vi "DAQmxTaskInfo.vi"(0 "task in":refnum<k21>) -> (1 "ChanType":i32, 2 "Name":refnum<k21>)   [LabVIEW 2010]
uses:
  Program Files/National Instruments/LabVIEW 2010/resource/objmgr/daqmx.rc
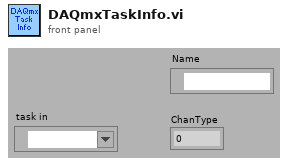
[diagram p1: front panel]
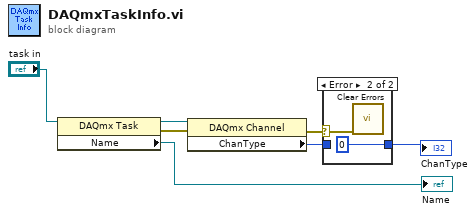
[diagram p0: block diagram]
diagram:
  n1 = property class="DAQmx Task"(reference="task in") -> (reference out=w3:refnum<k21>, error out=w1:errorcluster, "Name"=→"Name":refnum<k21>)  [unwired: 1 in]
  n2 = property class="DAQmx Channel"(reference=w3, error in=w1) -> (error out=w5:errorcluster, "ChanType"=w6:i32)  [unwired: 1 out]
  n3 = case shown="Error" w5 {
    selector: w5 -> [_ w10]
    tunnel: w6 -> [w8 _]
    tunnel: [w8 0 ("ChanType")] -> w7
    frame No Error {
    }
    frame Error {
      n4 = call <vilib>:"Clear Errors.vi"("error in (no error)"=w10) -> ()  [unwired: 6 in, 1 out]
    }
  }
  "ChanType" <- w7
